vi "DSF.Engine.Execution.Builder.Top.vi"(8 "error in (no error)":errorcluster, 11 "Builder in":refnum<class "DSF.Engine.Execution.Builder.lvclass">) -> (0 "error out":errorcluster, 3 "Builder out":refnum<class "DSF.Engine.Execution.Builder.lvclass">)   [LabVIEW 2016, in "DSF.Engine.lvlib" / "DSF.Engine.Execution.Builder.lvclass"]
uses:
  Builder/DSF.Engine.Execution.Builder.lvclass
  Builder/DSF.Engine.Execution.Builder.lvclass/DSF.Engine.Execution.Builder.ctl
  <vilib>/Platform/TimedLoop/XDataNode/timing_clust.ctl
  <vilib>/Platform/TimedLoop/XDataNode/nitl_modes.ctl
  <vilib>/Platform/TimedLoop/XDataNode/wakeup.ctl
  Cache/DSF.Engine.Memory.Cache.Framework.lvclass/DSF.Engine.Memory.Cache.Framework.ctl
  Memory.Cache/DSF.Engine.Memory.Cache.Plugin.lvclass/DSF.Engine.Memory.Cache.Plugin.ctl
  Memory.Cache/DSF.Engine.Memory.Cache.Transfer.lvclass/DSF.Engine.Memory.Cache.Transfer.ctl
  Memory.Pointer/DSF.Engine.Memory.Pointer.VS Channels.lvclass/DSF.Engine.Memory.Pointer.VS Channels.ctl
  Submodules/Memory Manager/Source/Classes/Pointer/Memory.Pointer.lvclass/Memory.Pointer.ctl
  DSF.Engine.Execution.Builder.Get FIFOs.vi
  Memory.Buffer/Methods/DSF.Engine.Memory.Buffer.Insert Channels.Preserve Value.vi
  DSF.Engine.Execution.Builder.Get VS Channel Buffer.vi
  DSF.Engine.Execution.Builder.Get Framework Cache.vi
  Memory.Cache/DSF.Engine.Memory.Cache.Framework.Get Plugin Cache.vi
  Memory.Cache/DSF.Engine.Memory.Cache.Plugin.Get Transfer Cache.vi
  Memory.Cache/DSF.Engine.Memory.Cache.Transfer.Get Channel Configuration.vi
  Memory.Cache/DSF.Engine.Memory.Cache.Transfer.Get VS Channels Pointer.vi
  DSF.Engine.Execution.Builder.Set VS Channel Buffer.vi
  Memory.Cache/DSF.Engine.Memory.Cache.Transfer.Get Buffer.vi
  Memory.Pointer/DSF.Engine.Memory.Pointer.VS Channels.Read.1D.vi
  Memory.Buffer/Methods/DSF.Engine.Memory.Buffer.Extract Channels.Preserve Value.vi
  Memory.Pointer/DSF.Engine.Memory.Pointer.VS Channels.Write.1D.vi
  Memory.Cache/DSF.Engine.Memory.Cache.Framework.Get Largest Count.All Types.vi
  Memory.Buffer/Methods/DSF.Engine.Memory.Buffer.Write.vi
  Memory.Buffer/Methods/DSF.Engine.Memory.Buffer.Write.1D.Bool.vi
  Memory.Buffer/Methods/DSF.Engine.Memory.Buffer.Write.1D.SGL.vi
  Memory.Buffer/Methods/DSF.Engine.Memory.Buffer.Write.1D.DBL.vi
  Memory.Buffer/Methods/DSF.Engine.Memory.Buffer.Write.1D.I8.vi
  Memory.Buffer/Methods/DSF.Engine.Memory.Buffer.Write.1D.I16.vi
  Memory.Buffer/Methods/DSF.Engine.Memory.Buffer.Write.1D.I32.vi
  Memory.Buffer/Methods/DSF.Engine.Memory.Buffer.Write.1D.I64.vi
  Memory.Buffer/Methods/DSF.Engine.Memory.Buffer.Write.1D.U8.vi
  Memory.Buffer/Methods/DSF.Engine.Memory.Buffer.Write.1D.U16.vi
  Memory.Buffer/Methods/DSF.Engine.Memory.Buffer.Write.1D.U32.vi
  Memory.Buffer/Methods/DSF.Engine.Memory.Buffer.Write.1D.U64.vi
  Memory.Cache/DSF.Engine.Memory.Cache.Framework.Get Plugin Caches.vi
  Memory.Cache/DSF.Engine.Memory.Cache.Plugin.Get Transfer Caches.vi
  Memory.Pointer/DSF.Engine.Memory.Pointer.VS Channels.Get Channel Count.vi
  Submodules/Memory Manager/Source/Classes/Pointer/Methods/Memory.Pointer.Read.vi
  Submodules/Memory Manager/Source/Classes/Pointer/Methods/Memory.Pointer.Read.Safe.1D.DBL.vi
  Memory.Buffer/Methods/DSF.Engine.Memory.Buffer.Read.vi
  Memory.Buffer/Methods/DSF.Engine.Memory.Buffer.Read.1D.Bool.vi
  Memory.Buffer/Methods/DSF.Engine.Memory.Buffer.Read.1D.SGL.vi
  Memory.Buffer/Methods/DSF.Engine.Memory.Buffer.Read.1D.DBL.vi
  Memory.Buffer/Methods/DSF.Engine.Memory.Buffer.Read.1D.I8.vi
  Memory.Buffer/Methods/DSF.Engine.Memory.Buffer.Read.1D.I16.vi
  Memory.Buffer/Methods/DSF.Engine.Memory.Buffer.Read.1D.I32.vi
  Memory.Buffer/Methods/DSF.Engine.Memory.Buffer.Read.1D.I64.vi
  Memory.Buffer/Methods/DSF.Engine.Memory.Buffer.Read.1D.U8.vi
  Memory.Buffer/Methods/DSF.Engine.Memory.Buffer.Read.1D.U16.vi
  Memory.Buffer/Methods/DSF.Engine.Memory.Buffer.Read.1D.U32.vi
  Memory.Buffer/Methods/DSF.Engine.Memory.Buffer.Read.1D.U64.vi
  Submodules/Memory Manager/Source/Classes/Pointer/Methods/Memory.Pointer.Write.vi
  Submodules/Memory Manager/Source/Classes/Pointer/Methods/Memory.Pointer.Write.Safe.1D.DBL.vi
  Memory.Cache/DSF.Engine.Memory.Cache.Plugin.Get Largest Count.All Types.vi
  Submodules/Memory Manager/Source/Classes/Pointer/Methods/Memory.Pointer.Write.Safe.1D.Bool.vi
  Submodules/Memory Manager/Source/Classes/Pointer/Methods/Memory.Pointer.Write.Safe.1D.SGL.vi
  Submodules/Memory Manager/Source/Classes/Pointer/Methods/Memory.Pointer.Write.Safe.1D.I8.vi
  Submodules/Memory Manager/Source/Classes/Pointer/Methods/Memory.Pointer.Write.Safe.1D.I16.vi
  Submodules/Memory Manager/Source/Classes/Pointer/Methods/Memory.Pointer.Write.Safe.1D.I32.vi
  Submodules/Memory Manager/Source/Classes/Pointer/Methods/Memory.Pointer.Write.Safe.1D.I64.vi
  Submodules/Memory Manager/Source/Classes/Pointer/Methods/Memory.Pointer.Write.Safe.1D.U8.vi
  Submodules/Memory Manager/Source/Classes/Pointer/Methods/Memory.Pointer.Write.Safe.1D.U16.vi
  Submodules/Memory Manager/Source/Classes/Pointer/Methods/Memory.Pointer.Write.Safe.1D.U32.vi
  Submodules/Memory Manager/Source/Classes/Pointer/Methods/Memory.Pointer.Write.Safe.1D.U64.vi
  Submodules/Memory Manager/Source/Classes/Pointer/Methods/Memory.Pointer.Read.Unsafe.1D.DBL.vi
  Submodules/Memory Manager/Source/Classes/Pointer/Methods/Memory.Pointer.Parameter Check.Null Pointer.vi
  Submodules/Memory Manager/Source/Classes/Pointer/Methods/Memory.Pointer.Parameter Check.Subset.Power of 2.vi
  Submodules/Memory Manager/Source/Classes/Pointer/Methods/Memory.Pointer.Read.Safe.1D.Bool.vi
  Submodules/Memory Manager/Source/Classes/Pointer/Methods/Memory.Pointer.Read.Safe.1D.SGL.vi
  Submodules/Memory Manager/Source/Classes/Pointer/Methods/Memory.Pointer.Read.Safe.1D.I8.vi
  Submodules/Memory Manager/Source/Classes/Pointer/Methods/Memory.Pointer.Read.Safe.1D.I16.vi
  Submodules/Memory Manager/Source/Classes/Pointer/Methods/Memory.Pointer.Read.Safe.1D.I32.vi
  Submodules/Memory Manager/Source/Classes/Pointer/Methods/Memory.Pointer.Read.Safe.1D.I64.vi
  Submodules/Memory Manager/Source/Classes/Pointer/Methods/Memory.Pointer.Read.Safe.1D.U8.vi
  Submodules/Memory Manager/Source/Classes/Pointer/Methods/Memory.Pointer.Read.Safe.1D.U16.vi
  Submodules/Memory Manager/Source/Classes/Pointer/Methods/Memory.Pointer.Read.Safe.1D.U32.vi
  Submodules/Memory Manager/Source/Classes/Pointer/Methods/Memory.Pointer.Read.Safe.1D.U64.vi
  Submodules/Memory Manager/Source/Classes/Pointer/Methods/Memory.Pointer.Write.Unsafe.1D.DBL.vi
  Memory.Cache/DSF.Engine.Memory.Cache.Transfer.Get Largest Count.All Types.vi
  Submodules/Memory Manager/Source/Classes/Pointer/Methods/Memory.Pointer.Write.Unsafe.1D.Bool.vi
  Submodules/Memory Manager/Source/Classes/Pointer/Methods/Memory.Pointer.Write.Unsafe.1D.SGL.vi
  Submodules/Memory Manager/Source/Classes/Pointer/Methods/Memory.Pointer.Write.Unsafe.1D.I8.vi
  Submodules/Memory Manager/Source/Classes/Pointer/Methods/Memory.Pointer.Write.Unsafe.1D.I16.vi
  Submodules/Memory Manager/Source/Classes/Pointer/Methods/Memory.Pointer.Write.Unsafe.1D.I32.vi
  Submodules/Memory Manager/Source/Classes/Pointer/Methods/Memory.Pointer.Write.Unsafe.1D.I64.vi
  Submodules/Memory Manager/Source/Classes/Pointer/Methods/Memory.Pointer.Write.Unsafe.1D.U8.vi
  Submodules/Memory Manager/Source/Classes/Pointer/Methods/Memory.Pointer.Write.Unsafe.1D.U16.vi
  Submodules/Memory Manager/Source/Classes/Pointer/Methods/Memory.Pointer.Write.Unsafe.1D.U32.vi
  Submodules/Memory Manager/Source/Classes/Pointer/Methods/Memory.Pointer.Write.Unsafe.1D.U64.vi
  Submodules/Memory Manager/Source/Classes/Pointer/Accessors/Get Address.vi
  Submodules/Memory Manager/Source/Classes/Pointer/Methods/Memory.Pointer.Errors.vi
  Submodules/Memory Manager/Source/Classes/Pointer/Methods/Memory.Pointer.Errors.Null Pointer.vi
  Submodules/Memory Manager/Source/Classes/Pointer/Methods/Memory.Pointer.Errors.Out of Bounds.vi
  Submodules/Memory Manager/Source/Classes/Pointer/Accessors/Get Size.vi
  Submodules/Memory Manager/Source/VIs/Memory.Count to Size.Power of 2.vi
  Submodules/Memory Manager/Source/Classes/Pointer/Methods/Memory.Pointer.Read.Unsafe.1D.Bool.vi
  Submodules/Memory Manager/Source/Classes/Pointer/Methods/Memory.Pointer.Read.Unsafe.1D.SGL.vi
  Submodules/Memory Manager/Source/Classes/Pointer/Methods/Memory.Pointer.Read.Unsafe.1D.I8.vi
  Submodules/Memory Manager/Source/Classes/Pointer/Methods/Memory.Pointer.Read.Unsafe.1D.I16.vi
  Submodules/Memory Manager/Source/Classes/Pointer/Methods/Memory.Pointer.Read.Unsafe.1D.I32.vi
  Submodules/Memory Manager/Source/Classes/Pointer/Methods/Memory.Pointer.Read.Unsafe.1D.I64.vi
  Submodules/Memory Manager/Source/Classes/Pointer/Methods/Memory.Pointer.Read.Unsafe.1D.U8.vi
  Submodules/Memory Manager/Source/Classes/Pointer/Methods/Memory.Pointer.Read.Unsafe.1D.U16.vi
  Submodules/Memory Manager/Source/Classes/Pointer/Methods/Memory.Pointer.Read.Unsafe.1D.U32.vi
  Submodules/Memory Manager/Source/Classes/Pointer/Methods/Memory.Pointer.Read.Unsafe.1D.U64.vi
  Submodules/Memory Manager/Source/Classes/Pointer/Methods/Memory.Pointer.Errors.Create Error.vi
  Submodules/Memory Manager/Source/Submodules/SEH/Source/VIs/Static Error Handling.Source Buffer.Write.String.vi
  Submodules/Memory Manager/Source/Classes/Pointer/Methods/Memory.Pointer.Errors.Write Pointer Size.vi
  Submodules/Memory Manager/Source/Submodules/SEH/Source/VIs/Static Error Handling.Source Buffer.Write.Numeric.Scalar.Base10.vi
  Submodules/Memory Manager/Source/Submodules/SEH/Source/VIs/Static Error Handling.Source Buffer.Write.Numeric.Scalar.Base10 (U64).vi
  Submodules/Memory Manager/Source/Submodules/SEH/Source/VIs/Static Error Handling.Error Cluster Constant.vi
  Submodules/Memory Manager/Source/Submodules/SEH/Source/VIs/Static Error Handling.Error Cluster Constant (256B).vi
  Submodules/Memory Manager/Source/Submodules/SEH/Source/VIs/Static Error Handling.Parameters.Status.Set.vi
  Submodules/Memory Manager/Source/Submodules/SEH/Source/VIs/Static Error Handling.Parameters.Code.Set.vi
  Submodules/Memory Manager/Source/Submodules/SEH/Source/VIs/Static Error Handling.Parameters.VI Source.Set.vi
  Submodules/Memory Manager/Source/Constants/Memory.Constants.vi
  Submodules/Memory Manager/Source/Constants/Memory.Constants.Library Name.vi
  Submodules/Memory Manager/Source/Classes/Pointer/Methods/Memory.Pointer.Errors.Get Info.vi
  Memory.Pointer/DSF.Engine.Memory.Pointer.VS Channels.lvclass
  C:/Git/Sourcetree/DSF/Source/Submodules/Memory Manager/Source/Classes/Pointer/Memory.Pointer.lvclass
  Buffer/DSF.Engine.Memory.Buffer.lvclass
  <vilib>/platform/TimedLoop/XDataNode/XDataNode.xnode
  <vilib>/Platform/TimedLoop/XDataNode/XDNodeRunTimeDep.lvlib
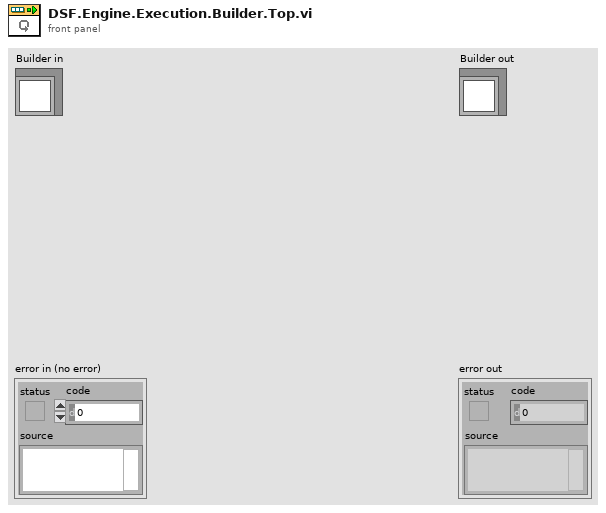
[diagram p1: front panel]
types:
  T1 = typedef "DSF.Shared.lvlib/DSF.Shared.RT Thread Parameters.ctl" = cluster{"Priority":i32, "Processor":i32}
  T2 = typedef "DSF.Engine.lvlib/DSF.Engine.Execution.Builder.lvclass/DSF.Engine.Execution.Builder.Type Buffers.ctl" = cluster{"Bool":bool[], "SGL":sgl[], "DBL":dbl[], "I8":i8[], "I16":i16[], "I32":i32[], "I64":i64[], "U8":u8[], "U16":u16[], "U32":u32[], "U64":u64[]}
  T3 = typedef "XDNodeRunTimeDep.lvlib/timing_clust.ctl" = cluster{"Expected End [f-1]":u64, "Actual End [f-1]":u64, "Finished Late? [f-1]":bool, "Expected End [i-1]":u64, "Actual End [i-1]":u64, "Finished Late? [i-1]":bool, "Expected Start [i]":u64, "Actual Start [i]":u64, "Expected Start [f]":u64, "Actual Start [f]":u64, "Source Name":string, "Structure Name":string, "Period":i64, "Deadline":i64, "Offset":i64, "Start":i64, "Priority":i32, "Timeout":i32, "Mode":T4, "Wakeup Reason":T5, "Error":errorcluster, "Source Type":string, "Secondary Source Type":string, "Global End Time":u64, "Global Start Time":u64, "Frame Duration":u64, "Iteration Duration":u64, "Assigned CPU":i32, "I/O Scan Engine Mode":u32}
  T4 = typedef "XDNodeRunTimeDep.lvlib/nitl_modes.ctl" = enum32{"No Change", "Process missed periods, maintain original phase", "Discard missed periods, maintain original phase", "Process missed periods, ignore original phase", "Discard missed periods, ignore original phase"}
  T5 = typedef "XDNodeRunTimeDep.lvlib/wakeup.ctl" = enum32{"Normal", "Aborted", "Asynchronous wakeup", "Timing source error", "Timed loop error", "Timeout"}
  T6 = typedef "DSF.Engine.lvlib/DSF.Engine.Execution.Builder.lvclass/DSF.Engine.Execution.Builder.Execution Settings.ctl" = cluster{"Command Timeout":i32, "Response Timeout":i32}
  T7 = typedef "DSF.Engine.lvlib/DSF.Engine.Execution.Builder.lvclass/DSF.Engine.Execution.Builder.Command Payload.ctl" = cluster{"Command":T8, "Plugin ID":i32, "Transfer ID":i32}
  T8 = typedef "DSF.Engine.lvlib/DSF.Engine.Execution.Builder.lvclass/DSF.Engine.Execution.Builder.Commands.ctl" = enum8{"Initialize", "Build", "Parse", "Shutdown"}
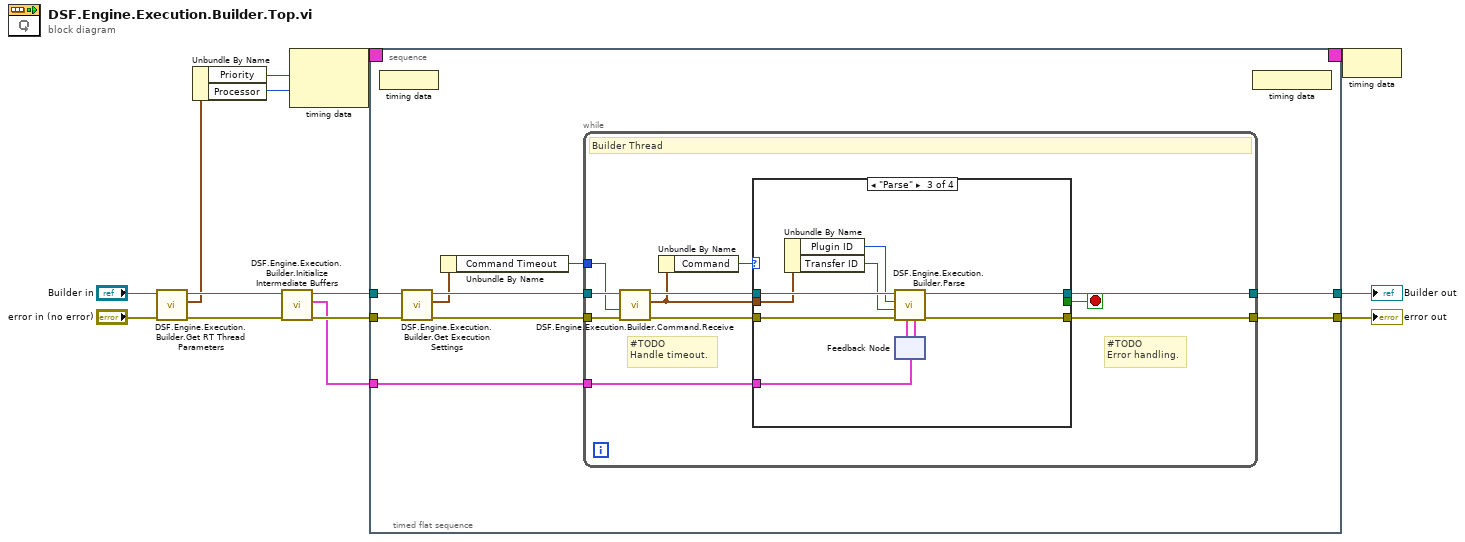
[diagram p0: block diagram]
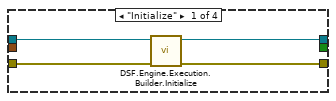
[diagram p2: hidden frame]
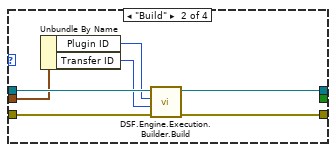
[diagram p3: hidden frame]
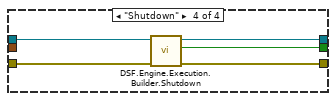
[diagram p4: hidden frame]
diagram:
  n1 = call "DSF.Engine.Execution.Builder.Get RT Thread Parameters.vi"("error in (no error)"="error in (no error)", "Builder in"="Builder in") -> ("error out"=w5:errorcluster, "RT Thread Parameters"=w1:T1, "Builder out"=w6:refnum<class "DSF.Engine.Execution.Builder.lvclass">)  [unwired: 7 in]
  n2 = Unbundle By Name(w1) -> ("Priority"=w10:i32, "Processor"=w9:i32)
  n3 = call "DSF.Engine.Execution.Builder.Initialize Intermediate Buffers.vi"("error in (no error)"=w5, "Builder in"=w6) -> ("error out"=w3:errorcluster, "Data Type Buffers"=w2:T2, "Builder out"=w4:refnum<class "DSF.Engine.Execution.Builder.lvclass">)  [unwired: 7 in]
  n4 = node-c288(w10, w9) -> (w14:T3)
  n5 = timed-sequence {
    timing: w14 -> [_]
    timing-out: [_] -> w13
    tunnel: [w19] -> w8
    tunnel: [w18] -> w7
    tunnel: w4 -> [w17]
    tunnel: w3 -> [w16]
    tunnel: w2 -> [w15]
    n6 = timed-flat-sequence {
      tunnel: [w24] -> w19
      tunnel: [w23] -> w18
      tunnel: w17 -> [w22]
      tunnel: w16 -> [w21]
      tunnel: w15 -> [w20]
      n7 = node-c288() -> ()  [unwired: 1 in]
      n8 = call "DSF.Engine.Execution.Builder.Get Execution Settings.vi"("error in (no error)"=w21, "Builder in"=w22) -> ("error out"=w26:errorcluster, "Execution Settings"=w25:T6, "Builder out"=w27:refnum<class "DSF.Engine.Execution.Builder.lvclass">)  [unwired: 7 in]
      n9 = Unbundle By Name(w25) -> ("Command Timeout"=w28:i32)
      n10 = while {
        tunnel: w27 -> [w41]
        tunnel: w26 -> [w40]
        tunnel: w28 -> [w39]
        tunnel: [w34] -> w24
        tunnel: [w33] -> w23
        tunnel: w20 -> [w31]
        stop <- w32 stop-if-true
        # "#TODO\nError handling."
        # "#TODO\nHandle timeout."
        # "Builder Thread"
        n11 = call "DSF.Engine.Execution.Builder.Command.Receive.vi"("error in (no error)"=w40, "timeout in ms (0)"=w39, "Builder in"=w41) -> ("error out"=w36:errorcluster, "Command"=w35:T7, "Builder out"=w37:refnum<class "DSF.Engine.Execution.Builder.lvclass">)  [unwired: 5 in, 1 out]
        n12 = Unbundle By Name(w35) -> ("Command"=w38:T8)
        n13 = case shown="\"Parse\"" w38 {
          tunnel: w37 -> [w42 w52 w62 w67]
          tunnel: w36 -> [w45 w51 w61 w66]
          tunnel: w35 -> [_ w48 w58 _]
          tunnel: [w44 w49 w59 w65] -> w34
          tunnel: [w43 w50 w60 w64] -> w33
          tunnel: [_ _ _ w63] -> w32
          tunnel: w31 -> [_ _ w55 _]
          frame "Initialize" {
            n14 = call "DSF.Engine.Execution.Builder.Initialize.vi"("error in (no error)"=w45, "Builder in"=w42) -> ("error out"=w43:errorcluster, "Builder out"=w44:refnum<class "DSF.Engine.Execution.Builder.lvclass">)  [unwired: 8 in]
          }
          frame "Build" {
            n15 = Unbundle By Name(w48) -> ("Plugin ID"=w47:i32, "Transfer ID"=w46:i32)
            n16 = call "DSF.Engine.Execution.Builder.Build.vi"("error in (no error)"=w51, "Transfer ID"=w46, "Plugin ID"=w47, "Builder in"=w52) -> ("error out"=w50:errorcluster, "Builder out"=w49:refnum<class "DSF.Engine.Execution.Builder.lvclass">)  [unwired: 6 in]
          }
          frame "Parse" {
            n17 = Unbundle By Name(w58) -> ("Plugin ID"=w56:i32, "Transfer ID"=w57:i32)
            n18 = feedback #1(w55) -> (w53:T2)
            n19 = call "DSF.Engine.Execution.Builder.Parse.vi"("Data Type Buffers in"=w53, "error in (no error)"=w61, "Transfer ID"=w57, "Plugin ID"=w56, "Builder in"=w62) -> ("error out"=w60:errorcluster, "Builder out"=w59:refnum<class "DSF.Engine.Execution.Builder.lvclass">, "Data Type Buffers out"=w54:T2)  [unwired: 4 in]
            n20 = feedback-in #1(w54) -> ()
          }
          frame "Shutdown" {
            n21 = call "DSF.Engine.Execution.Builder.Shutdown.vi"("error in (no error)"=w66, "Builder in"=w67) -> ("error out"=w64:errorcluster, "stop?"=w63:bool, "Builder out"=w65:refnum<class "DSF.Engine.Execution.Builder.lvclass">)  [unwired: 7 in]
          }
        }
      }
      n22 = node-c288() -> ()  [unwired: 1 out]
    }
  }
  "error out" <- w7
  "Builder out" <- w8
  n23 = node-c288(w13) -> ()
